vi "Open VacuumPlus (subVi).vi"(2 "error in (no error)":errorcluster) -> (0 "error out":errorcluster, 1 "standard output":string)   [LabVIEW 2016]
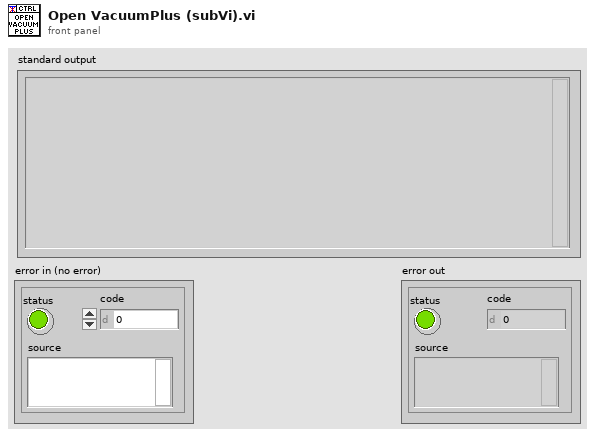
[diagram p1: front panel]
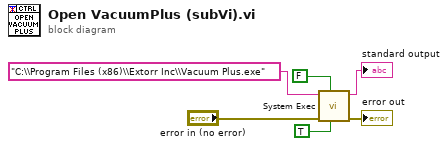
[diagram p0: block diagram]
diagram:
  n1 = call <vilib>:"System Exec.vi"("run minimized? (F)"=TRUE, "wait until completion? (T)"=FALSE, "error in (no error)"="error in (no error)", "command line"="C:\\Program Files (x86)\\Extorr Inc\\Vacuum Plus.exe") -> ("error out"=→"error out":errorcluster, "standard output"=→"standard output":string)  [unwired: 4 in, 2 out]
